vi "ConnectionDied.vi"(8 "error in (no error)":errorcluster, 10 "Connection":refnum<class "Connection.lvclass">, 11 "TcpServer in":refnum<class "TcpServer.lvclass">) -> (0 "error out":errorcluster, 3 "TcpServer out":refnum<class "TcpServer.lvclass">)   [LabVIEW 2022 SP3, in "TcpServer.lvlib" / "TcpServer.lvclass"]
uses:
  TcpServer.lvclass
  C:/Users/jakub/repos/gh/sw4sys/lv-tcp-server-sample/LoggingActor/Source/LoggingActor/LoggingActor/LoggingActor.lvclass
  TcpSocket/Source/TcpSocket/Connection/Connection.lvclass
  TcpSocket/Source/TcpSocket/Connection/Connection.lvclass/Connection.ctl
  TcpServer.lvclass/TcpServer.ctl
  LoggingActor/Source/LoggingActor/LoggingActor/LoggingActor.lvclass/LoggingActor.ctl
  TcpSocket/Source/TcpSocket/Connection/Read Address.vi
  TcpSocket/Source/TcpSocket/Connection/Read Port.vi
  TcpSocket/Source/TcpSocket/Connection/Read Connection.vi
  TcpSocket/Source/TcpSocket/Connection/Read ReadMode.vi
  TcpSocket/Source/TcpSocket/Connection/Read ReadTimeout.vi
  TcpSocket/Source/TcpSocket/Connection/Read WriteTimeout.vi
  LoggingActor/Source/LoggingActor/LoggingActor/Read Logger.vi
  Logger/Source/Logger/Logger.lvclass
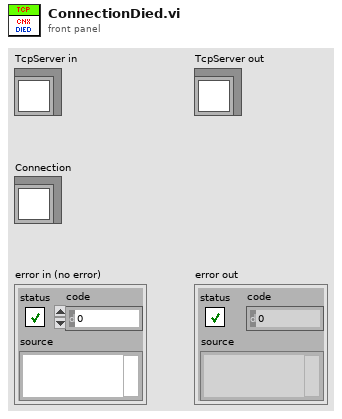
[diagram p1: front panel]
types:
  T1 = enum16{"Standard", "Buffered", "CRLF", "Immediate"}
  T2 = map{u64, refnum<class "Message Enqueuer.lvclass">}
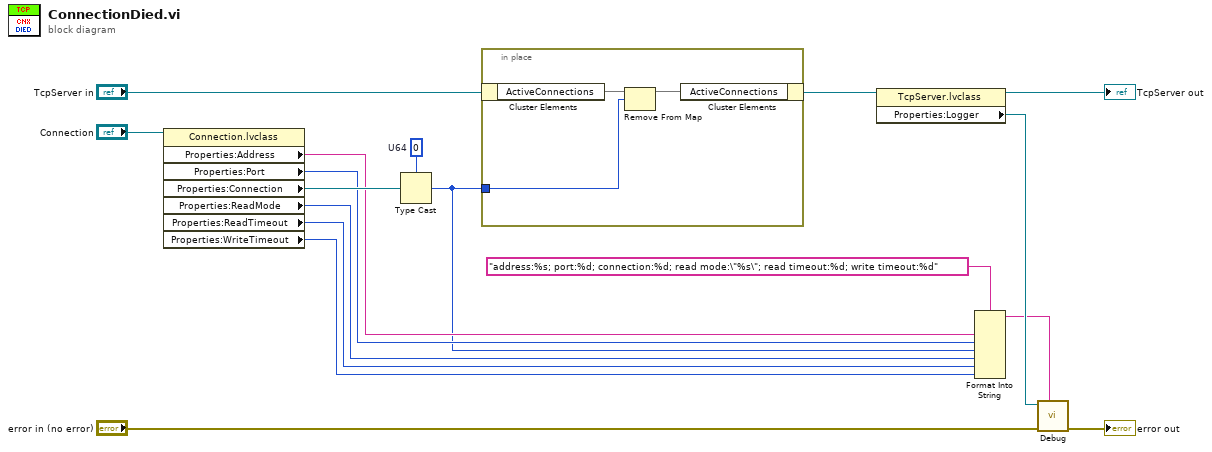
[diagram p0: block diagram]
diagram:
  w12 = u64 0  # U64
  n1 = property class="Connection.lvclass"(reference="Connection") -> ("Properties:Address"=w7:string, "Properties:Port"=w6:u16, "Properties:Connection"=w14:refnum<k5>, "Properties:ReadMode"=w4:T1, "Properties:ReadTimeout"=w3:i32, "Properties:WriteTimeout"=w2:i32)  [unwired: 1 in, 2 out]
  n2 = Type Cast(type=w12, x=w14) -> (*(type *) &x=w5:u64)
  n3 = in-place {
    in-place-border: w5 -> [w18]
    n4 = in-place-cluster #1("TcpServer in") -> ("ActiveConnections"=w20:T2)
    n5 = Remove From Map(10:w18, 11:w20) -> (3:w19:T2)  [unwired: 2 out]
    n6 = in-place-cluster #1("ActiveConnections"=w19) -> (w16:refnum<class "TcpServer.lvclass">)
  }
  n7 = property class="TcpServer.lvclass"(reference=w16) -> (reference out=→"TcpServer out":refnum<class "TcpServer.lvclass">, "Properties:Logger"=w9:refnum<class "Logger.lvclass">)  [unwired: 1 in, 1 out]
  n8 = Format Into String(format string="address:%s; port:%d; connection:%d; read mode:\"%s\"; read timeout:%d; write timeout:%d", w7, w6, w5, w4, w3, w2) -> (resulting string=w1:string)  [unwired: 2 in, 1 out]
  n9 = call-dynamic "Debug.vi"("Message"=w1, "error in (no error)"="error in (no error)", "Logger in"=w9) -> ("error out"=→"error out":errorcluster)  [unwired: 5 in, 1 out]
